vi "Str_To _UINT16.vi"(11 "Raw Data (string)":string) -> (3 "Data Out":u16[](array[numeric]))   [LabVIEW 2016]
panel:
  out "(hi.lo)":u16[](array[numeric])
  out "unsigned byte array":u8[](array[numeric]) format="%x"
  out "decimated array 2":u8[](array[numeric]) format="%x"
  out "decimated array":u8[](array[numeric]) format="%x"
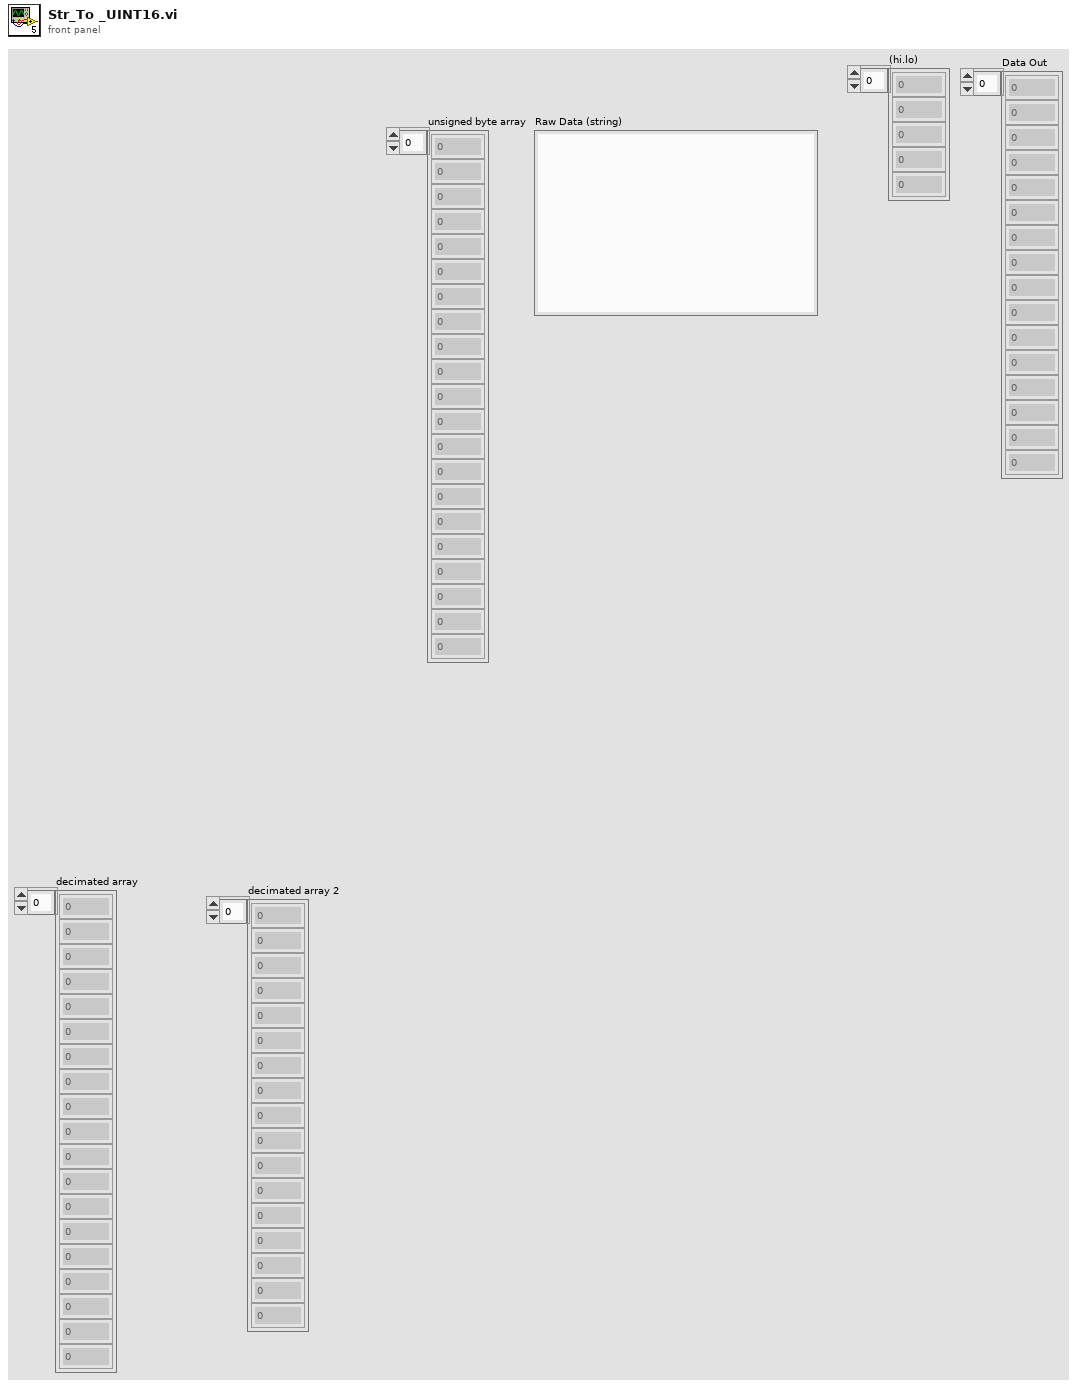
[diagram p1: front panel]
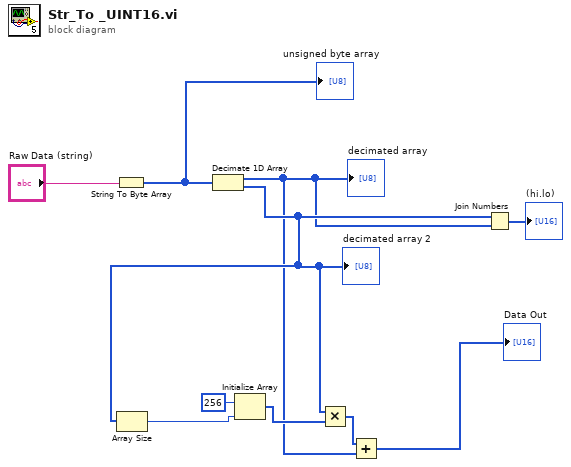
[diagram p0: block diagram]
diagram:
  n1 = String To Byte Array(string="Raw Data (string)") -> (unsigned byte array=w5:u8[])
  "unsigned byte array" <- w5
  n2 = Decimate 1D Array(w5) -> (w2:u8[], w3:u8[])
  "decimated array" <- w2
  "decimated array 2" <- w3
  n3 = Array Size(array=w3) -> (size(s)=w7:i32)
  n4 = Initialize Array(u16 256 ("element"), w7) -> (w8:u16[])
  n5 = Multiply(x=w3, y=w8) -> (x*y=w10:u16[])
  n6 = Add(x=w10, y=w2) -> (x+y=→"Data Out":u16[])
  n7 = Join Numbers(hi=w3, lo=w2) -> ((hi.lo)=→"(hi.lo)":u16[])
